vi "Remove ID.vi"(11 "id string":string) -> (2 "name":string, 3 "remaining id string":string)   [LabVIEW 2017, in "DSF Core.lvlib" / "Configuration Session.lvclass"]
uses:
  Configuration Session.lvclass
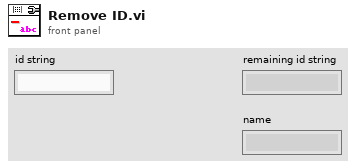
[diagram p1: front panel]
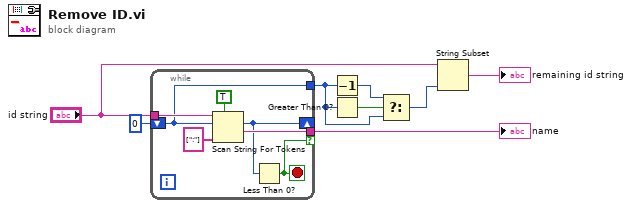
[diagram p0: block diagram]
diagram:
  n1 = while {
    tunnel: "id string" -> [w12]
    tunnel: [w13] -> w7 if=w10
    shift-right: [w11] -> _
    shift-left: 0 ("offset past token") -> [w9]
    tunnel: [w9] -> w3
    stop <- w10 stop-if-true
    n2 = Scan String For Tokens(5:TRUE ("allow empty tokens? (F)"), 6:string[] [":"] ("delimiters (\\s,\\t,\\r,\\n)"), 8:w9, 9:w12) -> (1:w13:string, 2:w11:i32)  [unwired: 2 in, 2 out]
    n3 = Less Than 0?(x=w11) -> (x < 0?=w10:bool)
  }
  "name" <- w7
  n4 = Decrement(x=w3) -> (x-1=w2:i32)
  n5 = Greater Than 0?(x=w3) -> (x > 0?=w1:bool)
  n6 = Select(t=w2, s=w1, f=w3) -> (s? t:f=w4:i32)
  n7 = String Subset(string="id string", length (rest)=w4) -> (substring=→"remaining id string":string)  [unwired: 1 in]
